vi "REACTOR__ADSORCION_MAIN.vi"() -> ()   [LabVIEW 2017]
doc: "Use this template to build a producer/consumer design pattern with events to produce queue items. Use this design pattern instead of the user interface event handler pattern for user interfaces when you want to execute code asynchronously in response to an event without slowing the user interface responsiveness."
uses:
  REACTOR_DATOS.ctl
  REACTOR_COMUNICACIONES.ctl
  SERIAL ALICATS/__s_TablaAlicats.ctl
  DISPLAY/Functions.ctl
  DISPLAY/User Event Data.ctl
  DISPLAY/Data Type.ctl
  REACTOR_CHANGE.ctl
  DISPLAY/PassedVars.ctl
  REACTOR_GLOBALES.vi
panel:
  out "MODO":bool
  out "ALICATS":T1=[["A", "NO", "aM0000013", "Air", "100", "ln/mn", "0.1", "0.11"], ["B", "NO", "aM0000014", "Air", "100", "ln/mn", "0.2", "0.22"], ["C", "NO", "aM0000015", "Air", "100", "ln/mn", "0.3", "0.33"], ["D", "NO", "aM0000016", "Air", "500", "ln/mn", "0.4", "0.44"]] caption="Alicats"
  out "st0":i32
  out "st1":i32
  in  "Tab Control":T2(tab)
  out "SPalcanzado":bool
  out "VALVE":bool
  out "Modo":string
  in  "Calor":bool
  in  "Frio":bool
  in  "Muestreo(s)":dbl=10.0
  in  "Comments":string="Añade aqui los comentarios...... y pincha fuera (sin teclear ENTER)"
  out "Ciclo(s)":i32
  out "Comments":string="Añade aqui los comentarios...... y pincha fuera (sin teclear ENTER)"
  in  "Programar":bool
  in  "Fin":bool
  in  "Auto":bool
  in  "Manual":bool
  in  "Valvula":bool
  in  "Parar":bool
  out "MF1":dbl caption="mL/min" format="%.2f"
  out "MF2":dbl caption="mL/min" format="%.2f"
  out "MF3":dbl caption="mL/min" format="%.2f"
  out "MF4":dbl caption="mL/min" format="%.2f"
  out "setTcalor":dbl caption="C" format="%.2f"
  out "Tcalor":dbl caption="C" format="%.2f"
  out "setTfrio":dbl caption="C" format="%.2f"
  out "Tfrio":dbl caption="C" format="%.2f"
  in  "Alicats":bool
  out "TIEMPO(min)":dbl format="%.2f"
  out "Lsample":bool
  out "StringA1":string
  out "C1":bool
  out "StringA2":string
  out "C2":bool
  out "StringA3":string
  out "C3":bool
  out "StringA4":string
  out "C4":bool
  out "XYTemp":cluster{dbl[], dbl[]}[](graph)
  out "Tcalor(C)":dbl format="%.1f"
  out "Tfrio(C)":dbl format="%.1f"
  out "XYFlows":cluster{dbl[], dbl[]}[](graph)
  out "Flujo4.":dbl format="%.2f"
  out "Flujo3.":dbl format="%.2f"
  out "Flujo2.":dbl format="%.2f"
  out "Flujo1.":dbl format="%.2f"
  in  "Completa":i32(listbox)
  in  "Secuencia":bool
  in  "Reducida":i32(listbox)
  in  "Pausa":bool
  in  "Saltar":bool
  in  "Max_t (s)":dbl=900.0 min=0.0 max=999.9 step=0.1 format="%.1f"
  in  "Delta_t (s)":dbl=60.0 min=0.0 max=999.9 step=0.1 format="%.1f"
  in  "Delta_T (C)":dbl=1.0 min=0.0 max=999.9 step=0.1 format="%.1f"
  out "Comunicaciones":T3={"Alicats"="ASRL6::INSTR", "Alic"=FALSE, "eValve"="ASRL6::INSTR", "eval"=FALSE, "Eurotherm"="ASRL6::INSTR", "euro"=FALSE, "Cell GAS"="ASRL6::INSTR", "cgas"=FALSE, "Cell H2S"="ASRL6::INSTR", "ch2s"=FALSE}
  out "Array":dbl[][](array[numeric])
  in  "Secuencia":string[](array[string])
  out "Datos":T4 {"a FSET4" format="%.2g"; "a FSET3" format="%.2g"; "a FSET2" format="%.2g"; "a FSET1" format="%.2g"; "a FLUJO4" format="%.2g"; "a FLUJO2" format="%.2g"; "a FLUJO1" format="%.2g"; "a FLUJO3" format="%.2g"; "eVAL_5" format="%.2g"; "TEMP_TH" format="%.2g"; "SET_TH" format="%.2g"; "TEMP_TC" format="%.2g"; "SET_TC" format="%.2g"; "TIEMPO" format="%.2g"}
  out "error out":errorcluster
  # "Entrada\n gases"
  # "PLANTA ADSORCION\n\nEnero 2023 Ver1.0 \na-sslcdms LV2017"
  # "CH4_40SCCM"
  # "Salida aire"
  # "N2_100SCCM"
  # "H2S_100SCCM"
  # "Salida\ngases"
  # "Entrada aire"
  # "H2S_10SCCM"
  # "Aire frio"
  # "Aire comprimido"
  # "Reactor"
  # "SERIE                          Controladores de flujo                     FLOWBUS"
  # "Condiciones de estabilidad en temperatura"
  # "Maxima variación \nde temperatura"
  # "en este intervalo \nde tiempo."
  # "Maximo tiempo posible \nsin alcanzar estabilidad"
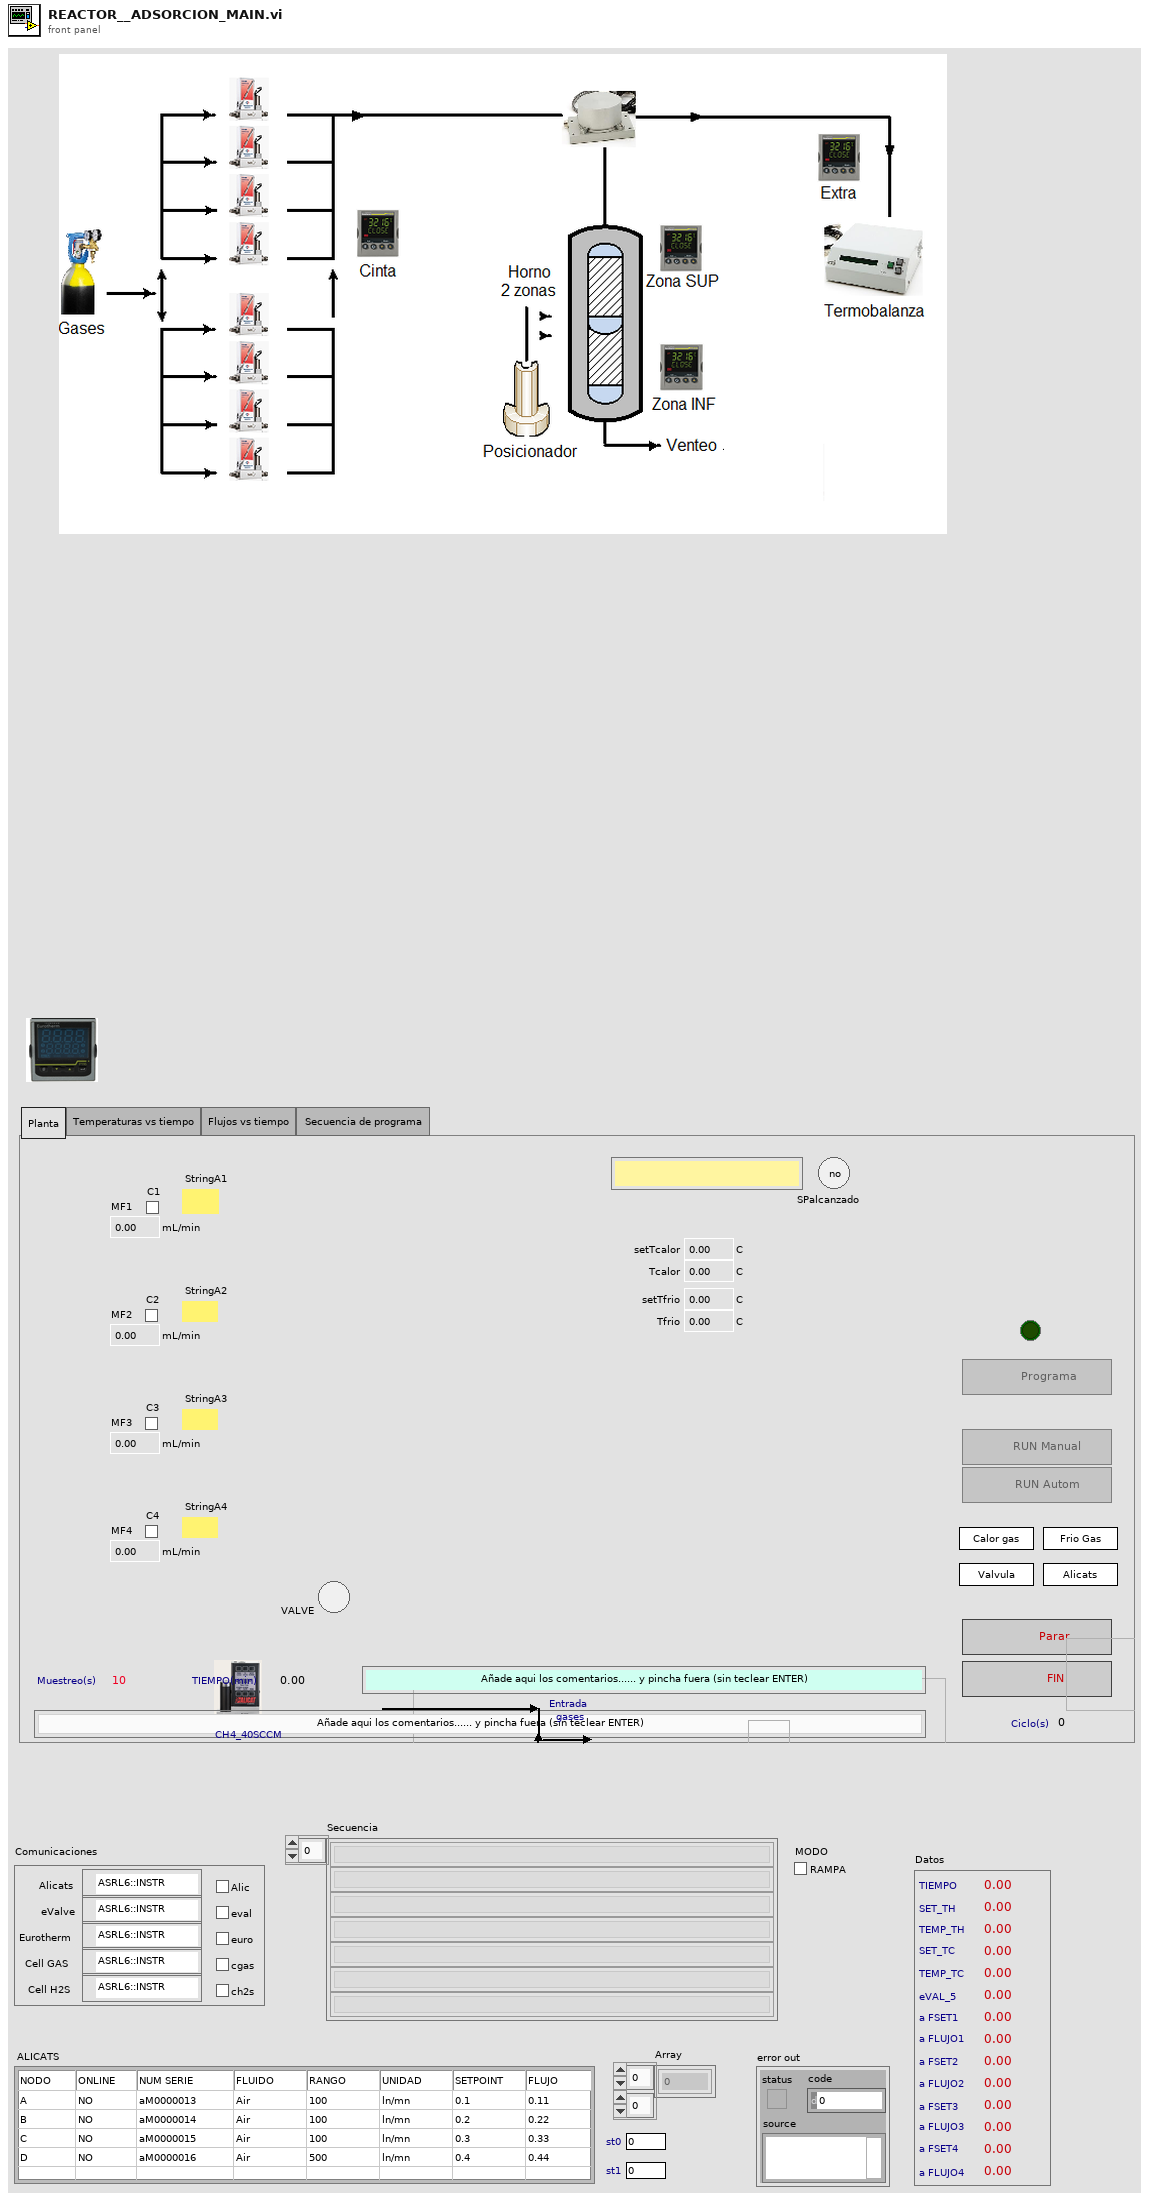
[diagram p1: front panel]
types:
  T1 = typedef "__s_TablaAlicats.ctl" = string[][]
  T2 = enum32{"Planta", "Temperaturas vs tiempo", "Flujos vs tiempo", "Secuencia de programa "}
  T3 = typedef "REACTOR_COMUNICACIONES.ctl" = cluster{"Alicats":refnum<visa-resource-name>, "Alic":bool, "eValve":refnum<visa-resource-name>, "eval":bool, "Eurotherm":refnum<visa-resource-name>, "euro":bool, "Cell GAS":refnum<visa-resource-name>, "cgas":bool, "Cell H2S":refnum<visa-resource-name>, "ch2s":bool}
  T4 = typedef "REACTOR_DATOS.ctl" = cluster{"TIEMPO":dbl, "SET_TH":dbl, "TEMP_TH":dbl, "SET_TC":dbl, "TEMP_TC":dbl, "eVAL_5":dbl, "a FSET1":dbl, "a FLUJO1":dbl, "a FSET2":dbl, "a FLUJO2":dbl, "a FSET3":dbl, "a FLUJO3":dbl, "a FSET4":dbl, "a FLUJO4":dbl}
  T5 = typedef "User Event Data.ctl" = cluster{"Data Type":T6, "Data":variant}
  T6 = typedef "Data Type.ctl" = enum16{"Init FP", "En/Dis FP Ctls", "Update FP", "Upd Status", "Upd Seq"}
  T7 = typedef "Functions.ctl" = enum16{"Initialize", "Run Man", "Run Auto", "Stop"}
  T8 = typedef "REACTOR_CHANGE.ctl" = enum16{"Default", "Continue", "Change Alicats", "Change Valve", "Change Calor", "Change Frio"}
  T9 = typedef "PassedVars.ctl" = dbl
  T10 = cluster{"Ch1":string, "Ch2":string, "Ch3":string, "Ch4":string}
  T11 = cluster{"Ch1":bool, "Ch2":bool, "Ch3":bool, "Ch4":bool}
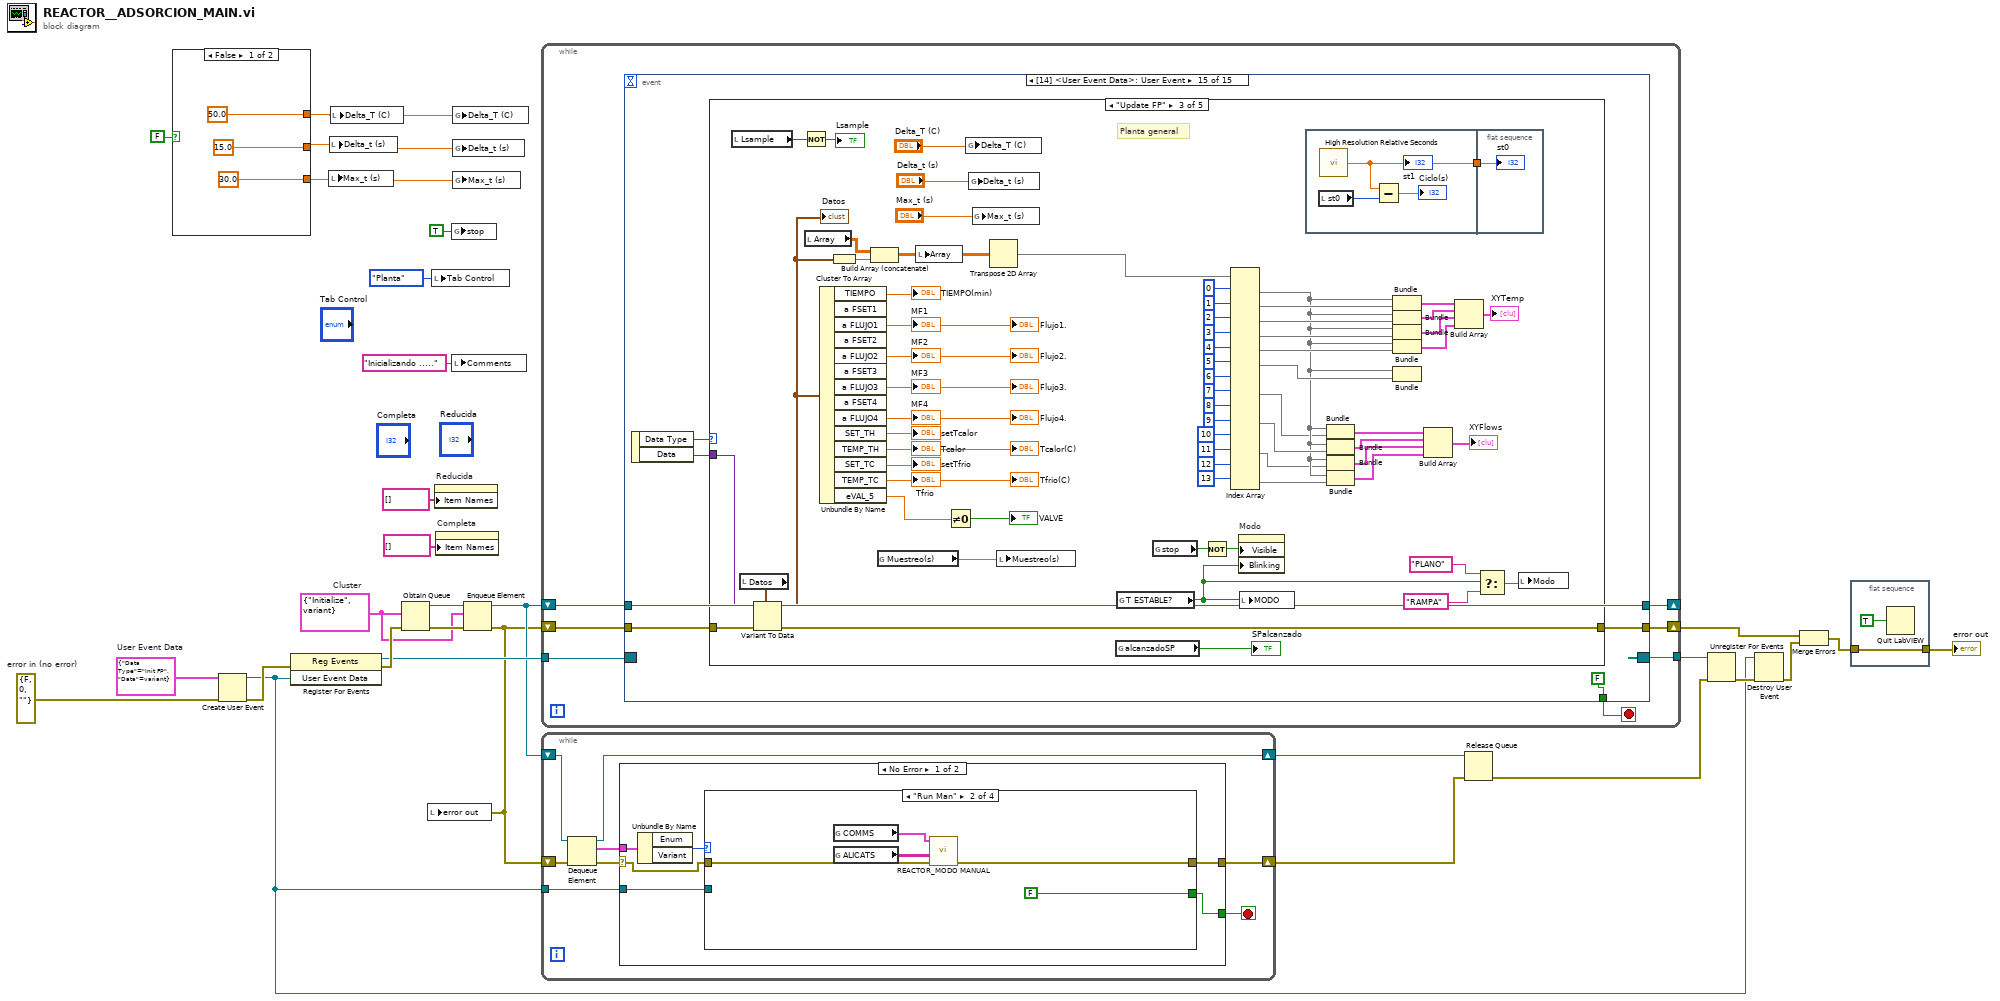
[diagram p0: block diagram]
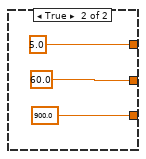
[diagram p2: hidden frame]
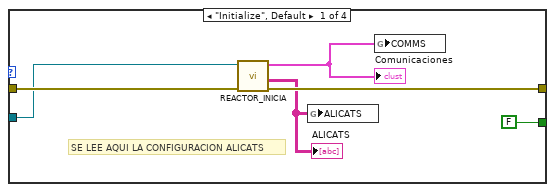
[diagram p3: hidden frame]
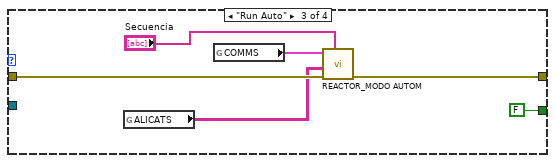
[diagram p4: hidden frame]
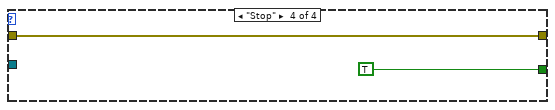
[diagram p5: hidden frame]
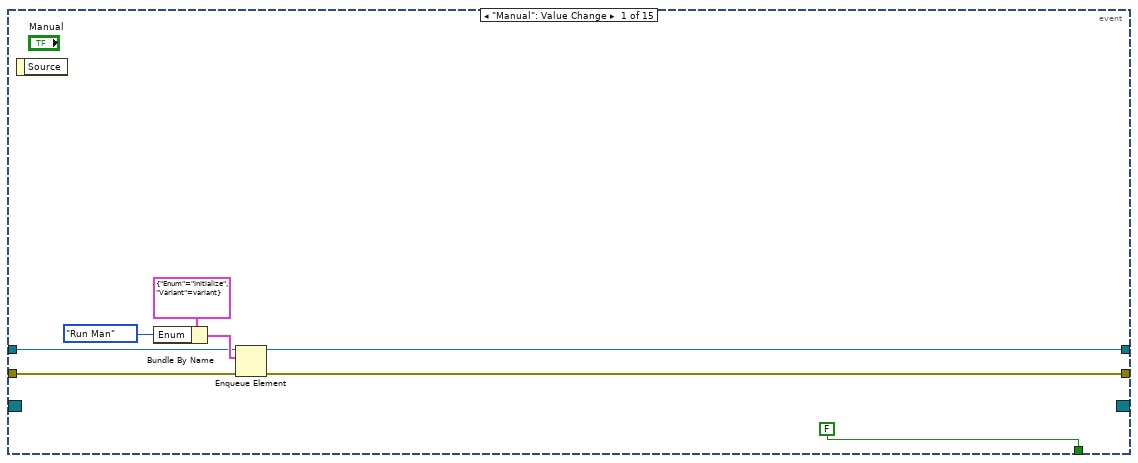
[diagram p7: hidden frame]
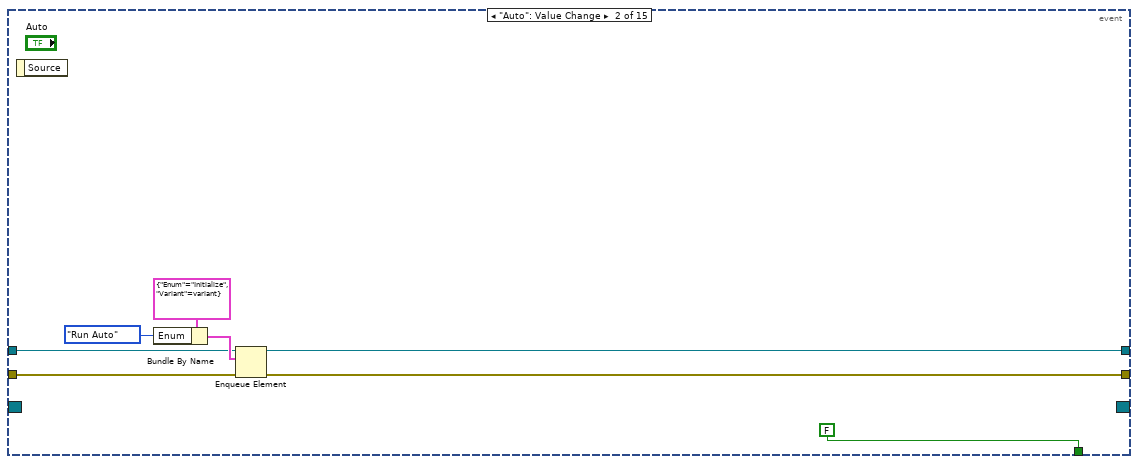
[diagram p8: hidden frame]
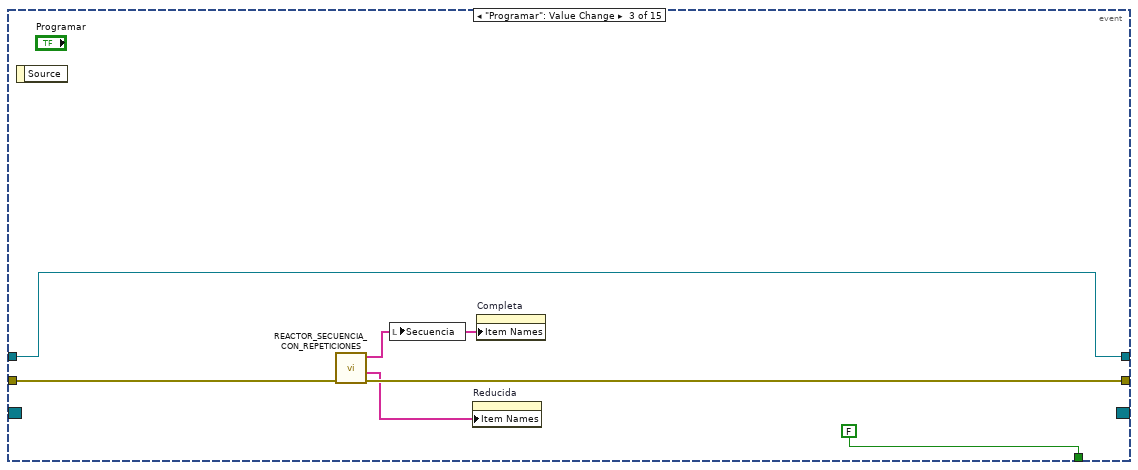
[diagram p9: hidden frame]
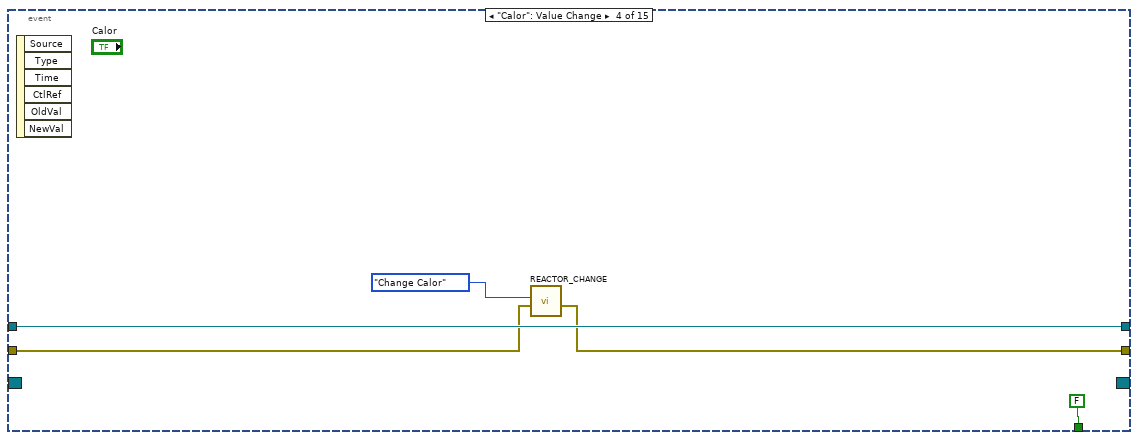
[diagram p10: hidden frame]
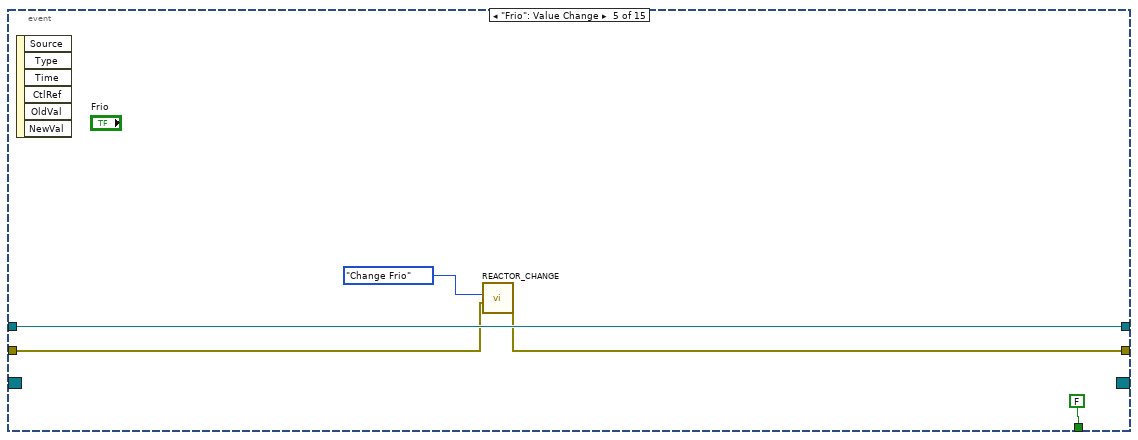
[diagram p11: hidden frame]
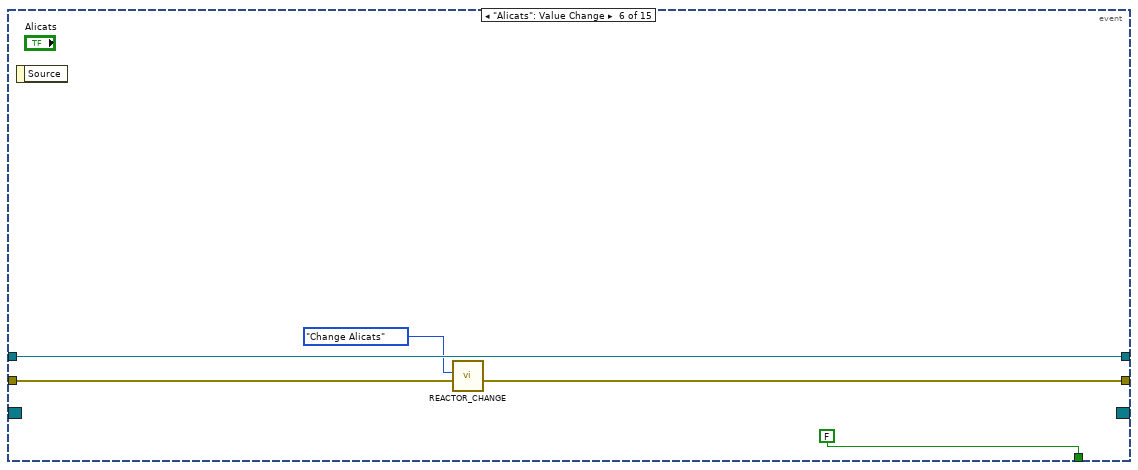
[diagram p12: hidden frame]
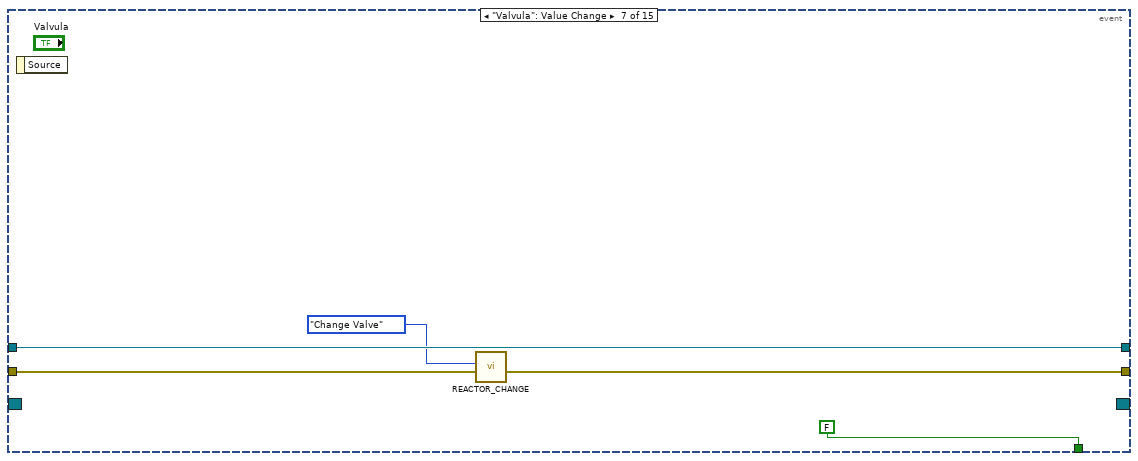
[diagram p13: hidden frame]
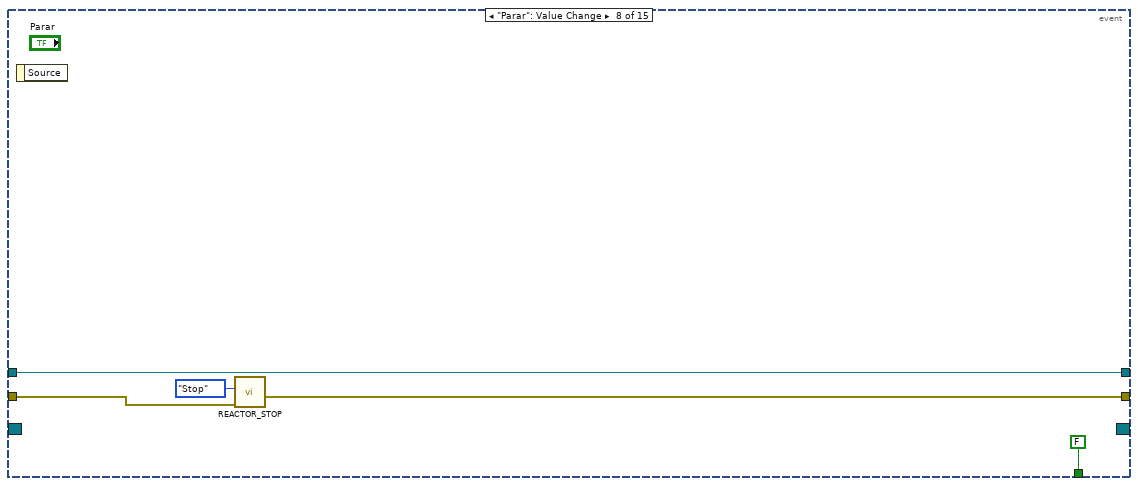
[diagram p14: hidden frame]
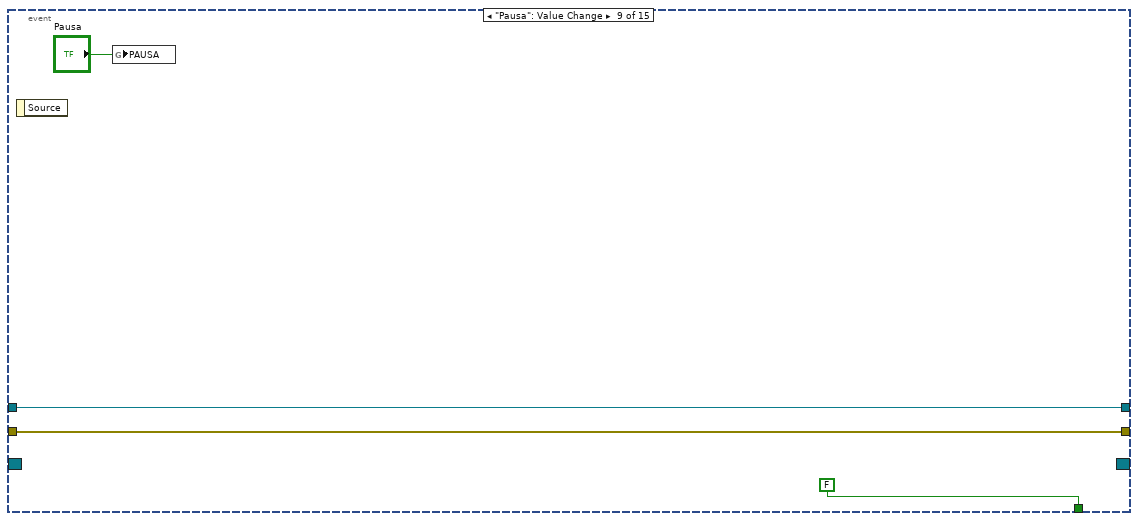
[diagram p15: hidden frame]
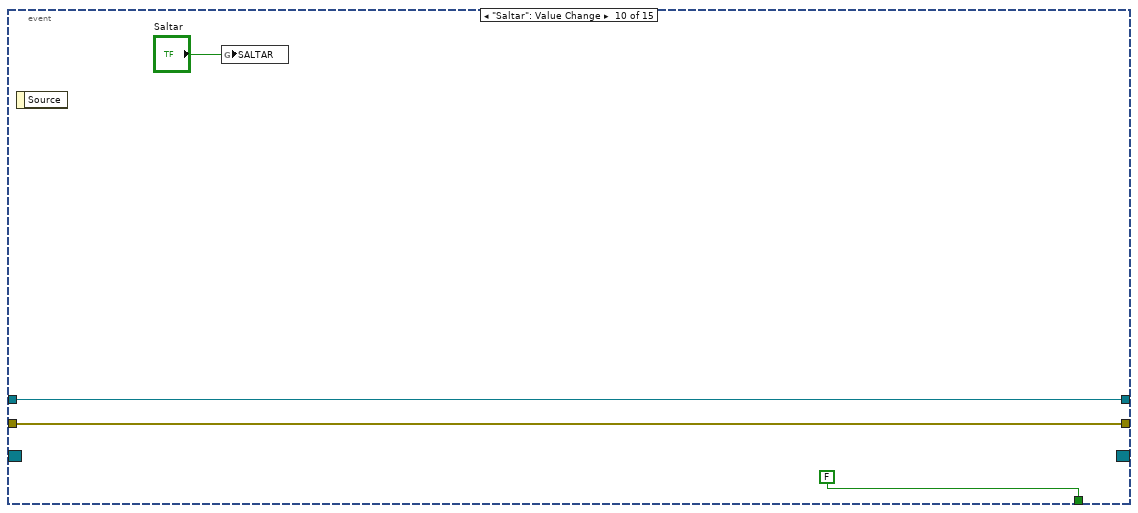
[diagram p16: hidden frame]
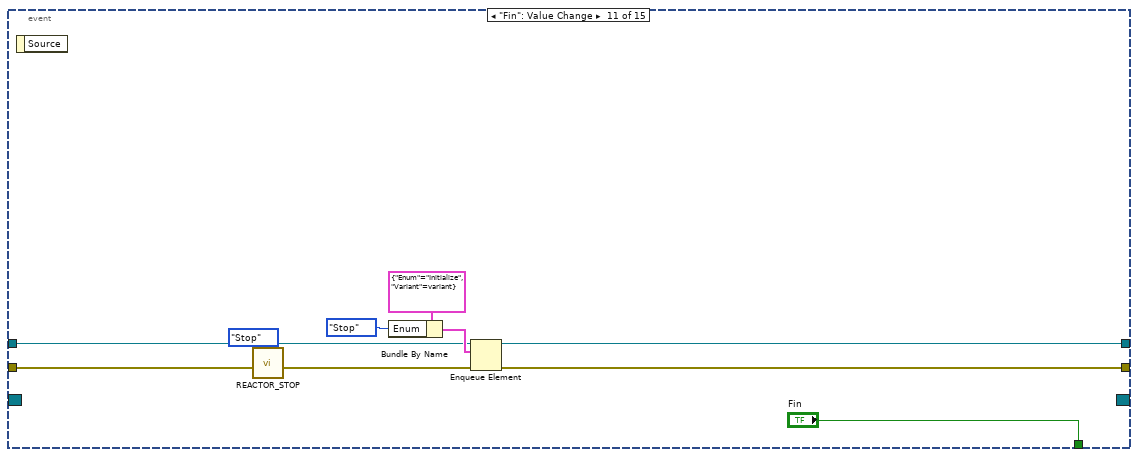
[diagram p17: hidden frame]
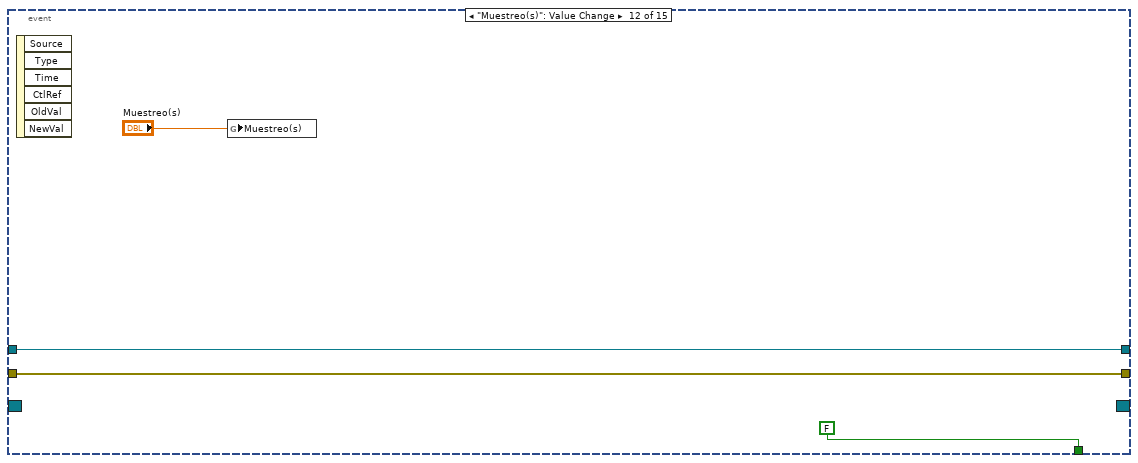
[diagram p18: hidden frame]
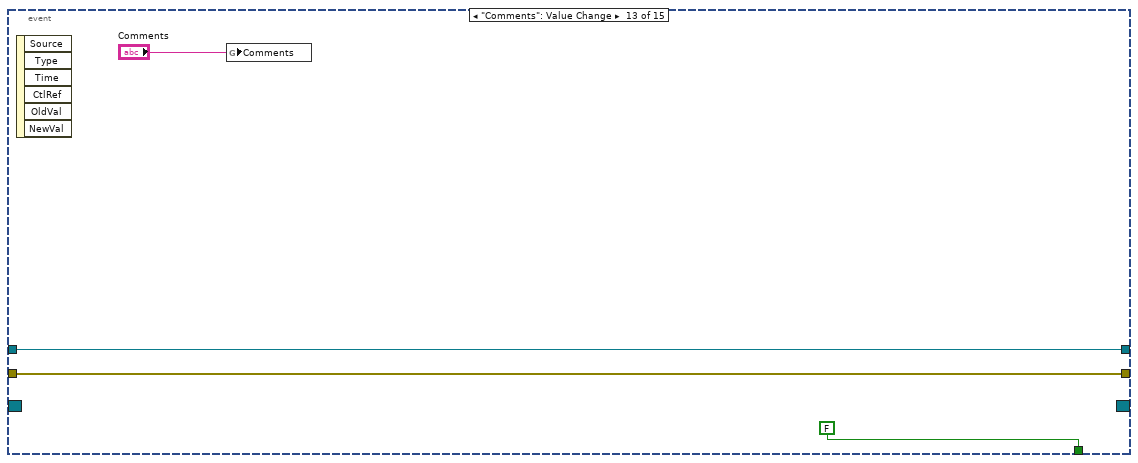
[diagram p19: hidden frame]
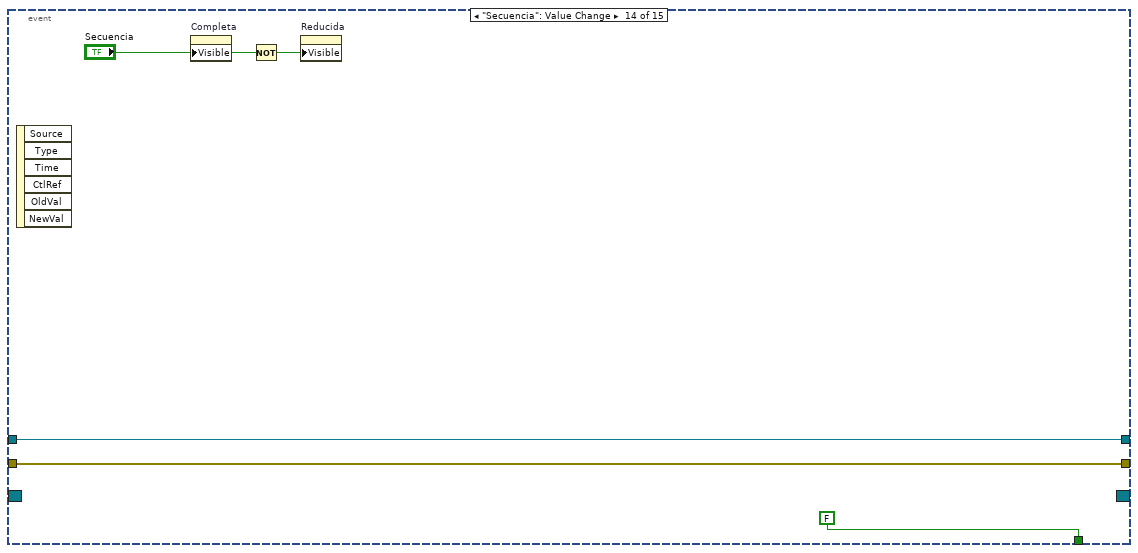
[diagram p20: hidden frame]
diagram:
  w16 = T5 {"Data Type"=enum."Init FP", "Data"=variant}  # User Event Data
  w8 = errorcluster {"status"=FALSE, "code"=0, "source"=""}  # error in (no error)
  w26 = cluster{"Enum":T7, "Variant":variant} {"Enum"=enum."Initialize", "Variant"=variant}  # Cluster
  n1 = case shown="False" FALSE {
    tunnel: [50.0 ("Delta_T (C)") 5.0 ("Delta_T (C)")] -> w6
    tunnel: [15.0 ("Delta_t (s)") 60.0 ("Delta_t (s)")] -> w5
    tunnel: [30.0 ("Max_t (s)") 900.0 ("Max_t (s)")] -> w4
    frame False {
    }
    frame True {
    }
  }
  n2 = Create User Event(user event datatype=w16, error in=w8) -> (user event=w13:refnum<user-event>, error out=w28:errorcluster)
  n3 = register-events(error in=w28, w13) -> (reference out=w18:refnum<event-registration>, error out=w29:errorcluster)  [unwired: 1 in]
  n4 = local write "Max_t (s)"(w4) -> ()
  n5 = local write "Delta_t (s)"(w5) -> ()
  n6 = local write "Delta_T (C)"(w6) -> ()
  n7 = Obtain Queue(element data type=w26, error in (no error)=w29) -> (queue out=w25:refnum<queue>, error out=w27:errorcluster)  [unwired: 3 in, 1 out]
  n8 = local write "Tab Control"(T2."Planta" ("Tab Control")) -> ()
  n9 = property on="Reducida" class="LstBox (strict)"("Item Names"=string[] []) -> ()  [unwired: 2 in, 2 out]
  n10 = property on="Completa" class="LstBox (strict)"("Item Names"=string[] []) -> ()  [unwired: 2 in, 2 out]
  n11 = global write "REACTOR_GLOBALES.vi" "stop"(TRUE ("stop")) -> ()
  n12 = local write "Comments"("Inicializando ....." ("String")) -> ()
  n13 = global write "REACTOR_GLOBALES.vi" "Delta_T (C)"(w6) -> ()
  n14 = global write "REACTOR_GLOBALES.vi" "Delta_t (s)"(w5) -> ()
  n15 = global write "REACTOR_GLOBALES.vi" "Max_t (s)"(w4) -> ()
  n16 = Enqueue Element(queue=w25, element=w26, error in (no error)=w27) -> (queue out=w15:refnum<queue>, error out=w14:errorcluster)  [unwired: 1 in, 1 out]
  n17 = local write "error out"(w14) -> ()
  n18 = while {
    shift-right: [w36] -> w21
    shift-left: w14 -> [w40]
    shift-right: [w41] -> _
    shift-left: w15 -> [w42]
    tunnel: w18 -> [w38]
    tunnel: [w37] -> w17
    stop <- w39 stop-if-true
    n19 = event shown="[14] <User Event Data>: User Event" {
      selector: w38 -> [_ _ _ _ _ _ _ _ _ _ _ _ _ _ _]
      dyn-events: [_ _ _ _ _ _ _ _ _ _ _ _ _ _ _] -> w37
      timeout: _ -> [_ _ _ _ _ _ _ _ _ _ _ _ _ _ _]
      tunnel: w42 -> [w45 w53 w59 w68 w73 w77 w81 w88 w92 w96 w102 w111 w115 w120 w122]
      tunnel: [w46 w54 w59 w68 w73 w77 w81 w88 w92 w96 w103 w111 w115 w120 w122] -> w41
      tunnel: w40 -> [w44 w52 w63 w67 w72 w76 w83 w87 w90 w94 w99 w109 w112 w116 w124]
      tunnel: [w47 w55 w62 w66 w71 w78 w82 w85 w90 w94 w104 w109 w112 w116 w123] -> w36
      tunnel: [FALSE ("Parar") FALSE ("Parar") FALSE ("Parar") FALSE ("Parar") FALSE ("Parar") FALSE ("Parar") FALSE ("Parar") FALSE ("Parar") FALSE ("Parar") FALSE ("Parar") "Fin" FALSE ("Parar") FALSE ("Parar") FALSE ("Parar") FALSE ("Parar")] -> w39
      event "Manual": Value Change {
        n20 = event-data() -> ()  [unwired: 1 in, 1 out]
        n21 = Bundle By Name(cluster=cluster{"Enum":T7, "Variant":variant} {"Enum"=enum."Initialize", "Variant"=variant} ("Cluster"), "Enum"=Functions."Run Man") -> (w48:cluster{"Enum":T7, "Variant":variant})
        n22 = Enqueue Element(queue=w45, element=w48, error in (no error)=w44) -> (queue out=w46:refnum<queue>, error out=w47:errorcluster)  [unwired: 1 in, 1 out]
      }
      event "Auto": Value Change {
        n23 = event-data() -> ()  [unwired: 1 in, 1 out]
        n24 = Bundle By Name(cluster=cluster{"Enum":T7, "Variant":variant} {"Enum"=enum."Initialize", "Variant"=variant} ("Cluster"), "Enum"=Functions."Run Auto") -> (w56:cluster{"Enum":T7, "Variant":variant})
        n25 = Enqueue Element(queue=w53, element=w56, error in (no error)=w52) -> (queue out=w54:refnum<queue>, error out=w55:errorcluster)  [unwired: 1 in, 1 out]
      }
      event "Programar": Value Change {
        n26 = event-data() -> ()  [unwired: 1 in, 1 out]
        n27 = call "REACTOR_SECUENCIA_CON_REPETICIONES.vi"("error in (no error)"=w63) -> ("error out"=w62:errorcluster, "Secuencia"=w60:string[], "Secuciclos"=w61:string[])  [unwired: 6 in, 2 out]
        n28 = local write "Secuencia"(w61) -> ()
        n29 = property on="Reducida" class="LstBox (strict)"("Item Names"=w60) -> ()  [unwired: 2 in, 2 out]
        n30 = property on="Completa" class="LstBox (strict)"("Item Names"=w61) -> ()  [unwired: 2 in, 2 out]
      }
      event "Calor": Value Change {
        n31 = event-data() -> ()  [unwired: 1 in, 6 out]
        n32 = call "REACTOR_CHANGE.vi"("error in (no error)"=w67, "Change"=REACTOR_CHANGE."Change Calor") -> ("error out"=w66:errorcluster)  [unwired: 8 in, 1 out]
      }
      event "Frio": Value Change {
        n33 = event-data() -> ()  [unwired: 1 in, 6 out]
        n34 = call "REACTOR_CHANGE.vi"("error in (no error)"=w72, "Change"=REACTOR_CHANGE."Change Frio") -> ("error out"=w71:errorcluster)  [unwired: 8 in, 1 out]
      }
      event "Alicats": Value Change {
        n35 = event-data() -> ()  [unwired: 1 in, 1 out]
        n36 = call "REACTOR_CHANGE.vi"("error in (no error)"=w76, "Change"=REACTOR_CHANGE."Change Alicats") -> ("error out"=w78:errorcluster)  [unwired: 8 in, 1 out]
      }
      event "Valvula": Value Change {
        n37 = event-data() -> ()  [unwired: 1 in, 1 out]
        n38 = call "REACTOR_CHANGE.vi"("error in (no error)"=w83, "Change"=REACTOR_CHANGE."Change Valve") -> ("error out"=w82:errorcluster)  [unwired: 8 in, 1 out]
      }
      event "Parar": Value Change {
        n39 = event-data() -> ()  [unwired: 1 in, 1 out]
        n40 = call "REACTOR_STOP.vi"("error in (no error)"=w87, "Stop"=enum16{"Continue", "Stop", "Default"}."Stop") -> ("error out"=w85:errorcluster)  [unwired: 8 in, 1 out]
      }
      event "Pausa": Value Change {
        n41 = event-data() -> ()  [unwired: 1 in, 1 out]
        n42 = global write "REACTOR_GLOBALES.vi" "PAUSA"("Pausa") -> ()
      }
      event "Saltar": Value Change {
        n43 = event-data() -> ()  [unwired: 1 in, 1 out]
        n44 = global write "REACTOR_GLOBALES.vi" "SALTAR"("Saltar") -> ()
      }
      event "Fin": Value Change {
        n45 = event-data() -> ()  [unwired: 1 in, 1 out]
        n46 = call "REACTOR_STOP.vi"("error in (no error)"=w99, "Stop"=enum16{"Continue", "Stop", "Default"}."Stop") -> ("error out"=w98:errorcluster)  [unwired: 8 in, 1 out]
        n47 = Bundle By Name(cluster=cluster{"Enum":T7, "Variant":variant} {"Enum"=enum."Initialize", "Variant"=variant} ("Cluster"), "Enum"=Functions."Stop") -> (w105:cluster{"Enum":T7, "Variant":variant})
        n48 = Enqueue Element(queue=w102, element=w105, error in (no error)=w98) -> (queue out=w103:refnum<queue>, error out=w104:errorcluster)  [unwired: 1 in, 1 out]
      }
      event "Muestreo(s)": Value Change {
        n49 = event-data() -> ()  [unwired: 1 in, 6 out]
        n50 = global write "REACTOR_GLOBALES.vi" "Muestreo(s)"("Muestreo(s)") -> ()
      }
      event "Comments": Value Change {
        n51 = event-data() -> ()  [unwired: 1 in, 6 out]
        n52 = global write "REACTOR_GLOBALES.vi" "Comments"("Comments") -> ()
      }
      event "Secuencia": Value Change {
        n53 = event-data() -> ()  [unwired: 1 in, 6 out]
        n54 = property on="Completa" class="LstBox (strict)"("Visible"="Secuencia") -> ()  [unwired: 2 in, 2 out]
        n55 = Not(x="Secuencia") -> (.not. x?=w118:bool)
        n56 = property on="Reducida" class="LstBox (strict)"("Visible"=w118) -> ()  [unwired: 2 in, 2 out]
      }
      event User Event {
        n57 = event-data() -> ("Data Type"=w126:T6, "Data"=w125:variant)  [unwired: 1 in]
        n58 = case shown="\"Update FP\"" w126 {
          tunnel: w125 -> [_ w153 w256 w267 w271]
          tunnel: w124 -> [w149 w156 w257 w266 w273]
          tunnel: [w149 w155 w241 w265 w272] -> w123
          frame "Init FP", Default {
            (unwired) "N2" ("String4")
            (unwired) "CO2" ("String3")
            (unwired) "AiR" ("String2")
            (unwired) "H2O" ("String1")
            w146 = cluster{dbl[], dbl[]}[] [] ("XYFlows")
            n59 = global read "REACTOR_GLOBALES.vi" "ALICATS_GASES"() -> (w133:T10)
            n60 = property on="Modo" class="Str"("Visible"=FALSE, "Blinking"=FALSE) -> ()  [unwired: 2 in, 2 out]
            n61 = Cluster To Array(cluster=w133) -> (array=w132:string[])
            n62 = Index Array(array=w132) -> (element #1=→"StringA1":string, element #2=→"StringA2":string, element #3=→"StringA3":string, element #4=→"StringA4":string)  [unwired: 4 in]
            n63 = global read "REACTOR_GLOBALES.vi" "T ESTABLE?"() -> (→"MODO":bool)
            n64 = global read "REACTOR_GLOBALES.vi" "VALVULA"() -> (w127:bool)
            n65 = global write "REACTOR_GLOBALES.vi" "Muestreo(s)"(T9 10.0 ("Lectura")) -> ()
            n66 = local write "VALVE"(w127) -> ()
            n67 = local write "XYFlows"(w146) -> ()
            n68 = global read "REACTOR_GLOBALES.vi" "ALICATS_NODES"() -> (w139:T11)
            n69 = local write "XYTemp"(w146) -> ()
            n70 = Cluster To Array(cluster=w139) -> (array=w138:bool[])
            n71 = local write "Comments"("Listo para comenzar" ("String")) -> ()
            n72 = Index Array(array=w138) -> (element #1=→"C1":bool, element #2=→"C2":bool, element #3=→"C3":bool, element #4=→"C4":bool)  [unwired: 4 in]
            n73 = property on="Datos" class="Clust (strict)"("Value"=T4 {"TIEMPO"=0.0, "SET_TH"=0.0, "TEMP_TH"=0.0, "SET_TC"=0.0, "TEMP_TC"=0.0, "eVAL_5"=0.0, "a FSET1"=0.0, "a FLUJO1"=0.0, "a FSET2"=0.0, "a FLUJO2"=0.0, "a FSET3"=0.0, "a FLUJO3"=0.0, "a FSET4"=0.0, "a FLUJO4"=0.0} ("Datos")) -> ()  [unwired: 2 in, 2 out]
            "Array" <- dbl[][] [] ("Array")
            "Modo" <- "Inicializando ....." ("Comments 2")
          }
          frame "En/Dis FP Ctls" {
            n74 = property on="Saltar" class="Bool"("Disabled"=u8 2) -> ()  [unwired: 2 in, 2 out]
            n75 = property on="Pausa" class="Bool (strict)"("Disabled"=u8 2) -> ()  [unwired: 2 in, 2 out]
            n76 = Variant To Data(error in=w156, type=0, Variant=w153) -> (data=w152:i32, error out=w155:errorcluster)
            n77 = case shown="1" w152 {
              frame 0, Default {
                # "Programa en pausa"
                n78 = property on="Saltar" class="Bool"("Disabled"=u8 0) -> ()  [unwired: 2 in, 2 out]
                n79 = property on="Pausa" class="Bool (strict)"("Disabled"=u8 0) -> ()  [unwired: 2 in, 2 out]
                n80 = property on="Calor" class="Bool"("Disabled"=u8 2) -> ()  [unwired: 2 in, 2 out]
                n81 = property on="Frio" class="Bool"("Disabled"=u8 2) -> ()  [unwired: 2 in, 2 out]
                n82 = property on="Alicats" class="Bool"("Disabled"=u8 2) -> ()  [unwired: 2 in, 2 out]
                n83 = property on="Valvula" class="Bool"("Disabled"=u8 2) -> ()  [unwired: 2 in, 2 out]
                n84 = property on="Programar" class="Bool"("Disabled"=u8 0) -> ()  [unwired: 2 in, 2 out]
                n85 = property on="Manual" class="Bool"("Disabled"=u8 0) -> ()  [unwired: 2 in, 2 out]
                n86 = property on="Auto" class="Bool"("Disabled"=u8 0) -> ()  [unwired: 2 in, 2 out]
                n87 = property on="Parar" class="Bool"("Disabled"=u8 0) -> ()  [unwired: 2 in, 2 out]
                n88 = property on="Fin" class="Bool"("Disabled"=u8 0) -> ()  [unwired: 2 in, 2 out]
              }
              frame 1 {
                # "Programa en manual"
                n89 = property on="Saltar" class="Bool"("Disabled"=u8 0) -> ()  [unwired: 2 in, 2 out]
                n90 = property on="Pausa" class="Bool (strict)"("Disabled"=u8 0) -> ()  [unwired: 2 in, 2 out]
                n91 = property on="Calor" class="Bool"("Disabled"=u8 0) -> ()  [unwired: 2 in, 2 out]
                n92 = property on="Frio" class="Bool"("Disabled"=u8 0) -> ()  [unwired: 2 in, 2 out]
                n93 = property on="Alicats" class="Bool"("Disabled"=u8 0) -> ()  [unwired: 2 in, 2 out]
                n94 = property on="Valvula" class="Bool"("Disabled"=u8 0) -> ()  [unwired: 2 in, 2 out]
                n95 = property on="Programar" class="Bool"("Disabled"=u8 2) -> ()  [unwired: 2 in, 2 out]
                n96 = property on="Manual" class="Bool"("Disabled"=u8 2) -> ()  [unwired: 2 in, 2 out]
                n97 = property on="Auto" class="Bool"("Disabled"=u8 2) -> ()  [unwired: 2 in, 2 out]
                n98 = property on="Parar" class="Bool"("Disabled"=u8 0) -> ()  [unwired: 2 in, 2 out]
                n99 = property on="Fin" class="Bool"("Disabled"=u8 0) -> ()  [unwired: 2 in, 2 out]
              }
              frame 2 {
                # "Programa en automatico"
                n100 = property on="Saltar" class="Bool"("Disabled"=u8 0) -> ()  [unwired: 2 in, 2 out]
                n101 = property on="Pausa" class="Bool (strict)"("Disabled"=u8 0) -> ()  [unwired: 2 in, 2 out]
                n102 = property on="Calor" class="Bool"("Disabled"=u8 2) -> ()  [unwired: 2 in, 2 out]
                n103 = property on="Frio" class="Bool"("Disabled"=u8 2) -> ()  [unwired: 2 in, 2 out]
                n104 = property on="Alicats" class="Bool"("Disabled"=u8 2) -> ()  [unwired: 2 in, 2 out]
                n105 = property on="Valvula" class="Bool"("Disabled"=u8 2) -> ()  [unwired: 2 in, 2 out]
                n106 = property on="Programar" class="Bool"("Disabled"=u8 2) -> ()  [unwired: 2 in, 2 out]
                n107 = property on="Manual" class="Bool"("Disabled"=u8 2) -> ()  [unwired: 2 in, 2 out]
                n108 = property on="Auto" class="Bool"("Disabled"=u8 2) -> ()  [unwired: 2 in, 2 out]
                n109 = property on="Parar" class="Bool"("Disabled"=u8 0) -> ()  [unwired: 2 in, 2 out]
                n110 = property on="Fin" class="Bool"("Disabled"=u8 0) -> ()  [unwired: 2 in, 2 out]
              }
            }
          }
          frame "Update FP" {
            # "Planta general"
            n111 = local read "Lsample"() -> (w236:bool)
            n112 = local read "Datos"() -> (w248:T4)
            n113 = Variant To Data(error in=w257, type=w248, Variant=w256) -> (data=w212:T4, error out=w241:errorcluster)
            "Datos" <- w212
            n114 = Not(x=w236) -> (.not. x?=→"Lsample":bool)
            n115 = local read "Array"() -> (w255:dbl[][])
            n116 = Unbundle By Name(w212) -> ("TIEMPO"=→"TIEMPO(min)":dbl, "a FLUJO1"=→"Flujo1." →"MF1":dbl, "a FLUJO2"=→"Flujo2." →"MF2":dbl, "a FLUJO3"=→"Flujo3." →"MF3":dbl, "a FLUJO4"=→"Flujo4." →"MF4":dbl, "SET_TH"=→"setTcalor":dbl, "TEMP_TH"=→"Tcalor(C)" →"Tcalor":dbl, "SET_TC"=→"setTfrio":dbl, "TEMP_TC"=→"Tfrio(C)" →"Tfrio":dbl, "eVAL_5"=w207:dbl)  [unwired: 4 out]
            n117 = Cluster To Array(cluster=w212) -> (array=w252:dbl[])
            n118 = Build Array (concatenate)(w255, w252) -> (w254:dbl[][])
            n119 = global read "REACTOR_GLOBALES.vi" "Muestreo(s)"() -> (w197:dbl)
            n120 = local write "Array"(w254) -> ()
            n121 = Not Equal To 0?(x=w207) -> (x != 0?=→"VALVE":bool)
            n122 = global write "REACTOR_GLOBALES.vi" "Delta_T (C)"("Delta_T (C)") -> ()
            n123 = global write "REACTOR_GLOBALES.vi" "Delta_t (s)"("Delta_t (s)") -> ()
            n124 = global write "REACTOR_GLOBALES.vi" "Max_t (s)"("Max_t (s)") -> ()
            n125 = Transpose 2D Array(2D array=w254) -> (transposed array=w253:dbl[][])
            n126 = local write "Muestreo(s)"(w197) -> ()
            n127 = global read "REACTOR_GLOBALES.vi" "alcanzadoSP"() -> (→"SPalcanzado":bool)
            n128 = global read "REACTOR_GLOBALES.vi" "T ESTABLE?"() -> (w191:bool)
            n129 = global read "REACTOR_GLOBALES.vi" "stop"() -> (w193:bool)
            n130 = Not(x=w193) -> (.not. x?=w192:bool)
            n131 = Index Array(array=w253, index (row) #1=0 ("index (row)"), index (row) #2=1 ("index (row)"), index (row) #3=2 ("index (row)"), index (row) #4=3 ("index (row)"), index (row) #5=4 ("index (row)"), index (row) #6=5 ("index (row)"), index (row) #7=6 ("index (row)"), index (row) #8=7 ("index (row)"), index (row) #9=8 ("index (row)"), index (row) #10=9 ("index (row)"), index (row) #11=10 ("index (row)"), index (row) #12=11 ("index (row)"), index (row) #13=12 ("index (row)"), index (row) #14=13 ("index (row)")) -> (element #1=w213:dbl[], element #2=w239:dbl[], element #3=w238:dbl[], element #4=w237:dbl[], element #5=w216:dbl[], element #6=w217:dbl[], element #8=w200:dbl[], element #10=w230:dbl[], element #12=w198:dbl[], element #14=w199:dbl[])  [unwired: 14 in, 4 out]
            n132 = property on="Modo" class="Str"("Visible"=w192, "Blinking"=w191) -> ()  [unwired: 2 in, 2 out]
            n133 = local write "MODO"(w191) -> ()
            n134 = flat-sequence {
              tunnel: [w259] -> w234
              tunnel: w234 -> [w261]
              frame #0 {
                n135 = local read "st0"() -> (w260:i32)
                n136 = call <vilib>:"High Resolution Relative Seconds.vi"() -> ("relative seconds"=w259:dbl)
                "st1" <- w259
                n137 = Subtract(x=w259, y=w260) -> (x-y=→"Ciclo(s)":dbl)
              }
              frame #1 {
                "st0" <- w261
              }
            }
            n138 = Bundle(w213, w200) -> (w247:cluster{dbl[], dbl[]})  [unwired: 1 in]
            n139 = Bundle(w213, w230) -> (w246:cluster{dbl[], dbl[]})  [unwired: 1 in]
            n140 = Bundle(w213, w198) -> (w245:cluster{dbl[], dbl[]})  [unwired: 1 in]
            n141 = Bundle(w213, w199) -> (w244:cluster{dbl[], dbl[]})  [unwired: 1 in]
            n142 = Bundle(w213, w239) -> (w250:cluster{dbl[], dbl[]})  [unwired: 1 in]
            n143 = Bundle(w213, w238) -> (w251:cluster{dbl[], dbl[]})  [unwired: 1 in]
            n144 = Bundle(w213, w237) -> (w242:cluster{dbl[], dbl[]})  [unwired: 1 in]
            n145 = Bundle(w213, w216) -> (w240:cluster{dbl[], dbl[]})  [unwired: 1 in]
            n146 = Bundle(w213, w217) -> ()  [unwired: 1 in, 1 out]
            n147 = Build Array(w247, w246, w245, w244) -> (→"XYFlows":cluster{dbl[], dbl[]}[])
            n148 = Build Array(w250, w251, w242, w240) -> (→"XYTemp":cluster{dbl[], dbl[]}[])
            n149 = Select(t="PLANO" ("Comments 2"), s=w191, f="RAMPA" ("Comments 2")) -> (s? t:f=w195:string)
            n150 = local write "Modo"(w195) -> ()
          }
          frame "Upd Status" {
            n151 = Variant To Data(error in=w266, type=" ", Variant=w267) -> (data=→"Comments":string, error out=w265:errorcluster)
            n152 = global read "REACTOR_GLOBALES.vi" "PAUSA"() -> (w262:bool)
            n153 = property on="Pausa" class="Bool (strict)"("Blinking"=w262) -> ()  [unwired: 2 in, 2 out]
          }
          frame "Upd Seq" {
            n154 = Variant To Data(error in=w273, type=0, Variant=w271) -> (data=w269:i32, error out=w272:errorcluster)
            n155 = Subtract(x=w269, y=4) -> (x-y=w270:i32)
            n156 = property on="Completa" class="LstBox (strict)"("Value (Signaling)"=w269) -> ()  [unwired: 2 in, 2 out]
            n157 = property on="Completa" class="LstBox (strict)"("Top Row"=w270) -> ()  [unwired: 2 in, 2 out]
          }
        }
      }
    }
  }
  n158 = while {
    shift-right: [w280] -> w20
    shift-left: w15 -> [w282]
    shift-right: [w276] -> w19
    shift-left: w14 -> [w281]
    tunnel: w13 -> [w275]
    stop <- w278 stop-if-true
    n159 = Dequeue Element(queue=w282, error in (no error)=w281) -> (queue out=w280:refnum<queue>, element=w277:cluster{"Enum":T7, "Variant":variant}, error out=w279:errorcluster)  [unwired: 1 in, 1 out]
    n160 = case shown="No Error" w279 {
      selector: w279 -> [w286 w308]
      tunnel: [w284 _] -> w278
      tunnel: w277 -> [w288 _]
      tunnel: [w285 w308] -> w276
      tunnel: w275 -> [w283 _]
      frame No Error {
        n161 = Unbundle By Name(w288) -> ("Enum"=w287:T7)  [unwired: 1 out]
        n162 = case shown="\"Run Man\"" w287 {
          tunnel: w286 -> [w293 w298 w304 w306]
          tunnel: [w292 w297 w303 w306] -> w285
          tunnel: [FALSE FALSE FALSE TRUE] -> w284
          tunnel: w283 -> [w291 _ _ _]
          frame "Initialize", Default {
            # "SE LEE AQUI LA CONFIGURACION ALICATS"
            n163 = call "REACTOR_INICIA.vi"("error in (no error)"=w293, "User event"=w291) -> ("error out"=w292:errorcluster, "ALICATS out"=w289:T1, "COMMS"=w290:T3)  [unwired: 7 in]
            "Comunicaciones" <- w290
            "ALICATS" <- w289
            n164 = global write "REACTOR_GLOBALES.vi" "ALICATS"(w289) -> ()
            n165 = global write "REACTOR_GLOBALES.vi" "COMMS"(w290) -> ()
          }
          frame "Run Man" {
            n166 = global read "REACTOR_GLOBALES.vi" "COMMS"() -> (w296:T3)
            n167 = global read "REACTOR_GLOBALES.vi" "ALICATS"() -> (w295:T1)
            n168 = call "REACTOR_MODO MANUAL.vi"("error in (no error)"=w298, "ALICATS"=w295, "Comms"=w296) -> ("error out"=w297:errorcluster)  [unwired: 8 in]
          }
          frame "Run Auto" {
            n169 = global read "REACTOR_GLOBALES.vi" "ALICATS"() -> (w300:T1)
            n170 = global read "REACTOR_GLOBALES.vi" "COMMS"() -> (w301:T3)
            n171 = call "REACTOR_MODO AUTOM.vi"("Secuencia"="Secuencia", "error in (no error)"=w304, "ALICATS"=w300, "Comms"=w301) -> ("error out"=w303:errorcluster)  [unwired: 7 in]
          }
          frame "Stop" {
          }
        }
      }
      frame Error {
      }
    }
  }
  n172 = Release Queue(queue=w20, error in (no error)=w19) -> (error out=w22:errorcluster)  [unwired: 1 in, 2 out]
  n173 = Unregister For Events(event registration refnum=w17, error in=w22) -> (error out=w23:errorcluster)
  n174 = Destroy User Event(user event=w13, error in=w23) -> (error out=w24:errorcluster)
  n175 = Merge Errors(w21, w24) -> (w11:errorcluster)
  n176 = flat-sequence {
    tunnel: w11 -> [w310]
    tunnel: [w310] -> w10
    frame #0 {
      n177 = Quit LabVIEW(quit? (T)=TRUE) -> ()
    }
  }
  "error out" <- w10
